vi "prepost.vi"(6 "What to call":enum16{"nothing", "pre-build", "post-build"}(ring), 7 "Post-build parameters":T1, 8 "error in (no error)":errorcluster, 11 "Build Parameters in":T2={"Build File"=path "", "File Format Version"=0, "Build Parameters v0.0"={"Project Root"=path "", "Build Root"=path "", "Source Root"=path "", "Namespace"="", "Overwrite Existing Files?"=FALSE, "Top Level VIs"=[], "Dynamic VIs"=[], "Exclude Lib Dirs from Build (None)"=[], "Destinations"=[]}, "Extra Parameters v1.0"={"Log File"=path "", "Include Hidden VIs"=FALSE, "Include Help Files"=FALSE, "Help File Dir"=path "", "Include Shared Libs"=TRUE, "Shared Lib Dir"=path "", "Include External Subrs"=TRUE, "External Subr Dir"=path "", "Support Files"=[], "EXE Icon File"=path "", "NewBuildRootDir"=FALSE, "UnsavedChangesMsgBox"=FALSE, "Ambiguous VIs Dest Dir"=path "", "Pre-build VI"=path "", "Post-build VI"=path "", "Revision File"=path "", "Version VI Name"="", "Version Ctrl Name"="", "Default Password"="", "RemovePolyVIsAndTDs"=FALSE, "Call-Back VIs"=[], "Allow CBVI & BH overlap"=FALSE, "Namespace convention"=enum."OpenG (suffix)", "Exe.AppFlags"=0, "Exe.LVRT Res Flags"=0}, "VI Property Specs"=[]} {"File Format Version" format="%.0x"; "Extra Parameters v1.0"."Exe.LVRT Res Flags" format="%.0x"; "Extra Parameters v1.0"."Exe.AppFlags" format="%.0x"}) -> (0 "error out":errorcluster, 1 "error type (fatal)":enum16{"fatal", "non-fatal", "warning"}(ring), 3 "Build Parameters in 2":T2={"Build File"=path "", "File Format Version"=0, "Build Parameters v0.0"={"Project Root"=path "", "Build Root"=path "", "Source Root"=path "", "Namespace"="", "Overwrite Existing Files?"=FALSE, "Top Level VIs"=[], "Dynamic VIs"=[], "Exclude Lib Dirs from Build (None)"=[], "Destinations"=[]}, "Extra Parameters v1.0"={"Log File"=path "", "Include Hidden VIs"=FALSE, "Include Help Files"=FALSE, "Help File Dir"=path "", "Include Shared Libs"=TRUE, "Shared Lib Dir"=path "", "Include External Subrs"=TRUE, "External Subr Dir"=path "", "Support Files"=[], "EXE Icon File"=path "", "NewBuildRootDir"=FALSE, "UnsavedChangesMsgBox"=FALSE, "Ambiguous VIs Dest Dir"=path "", "Pre-build VI"=path "", "Post-build VI"=path "", "Revision File"=path "", "Version VI Name"="", "Version Ctrl Name"="", "Default Password"="", "RemovePolyVIsAndTDs"=FALSE, "Call-Back VIs"=[], "Allow CBVI & BH overlap"=FALSE, "Namespace convention"=enum."OpenG (suffix)", "Exe.AppFlags"=0, "Exe.LVRT Res Flags"=0}, "VI Property Specs"=[]} {"File Format Version" format="%.0x"; "Extra Parameters v1.0"."Exe.LVRT Res Flags" format="%.0x"; "Extra Parameters v1.0"."Exe.AppFlags" format="%.0x"})   [LabVIEW 2009]
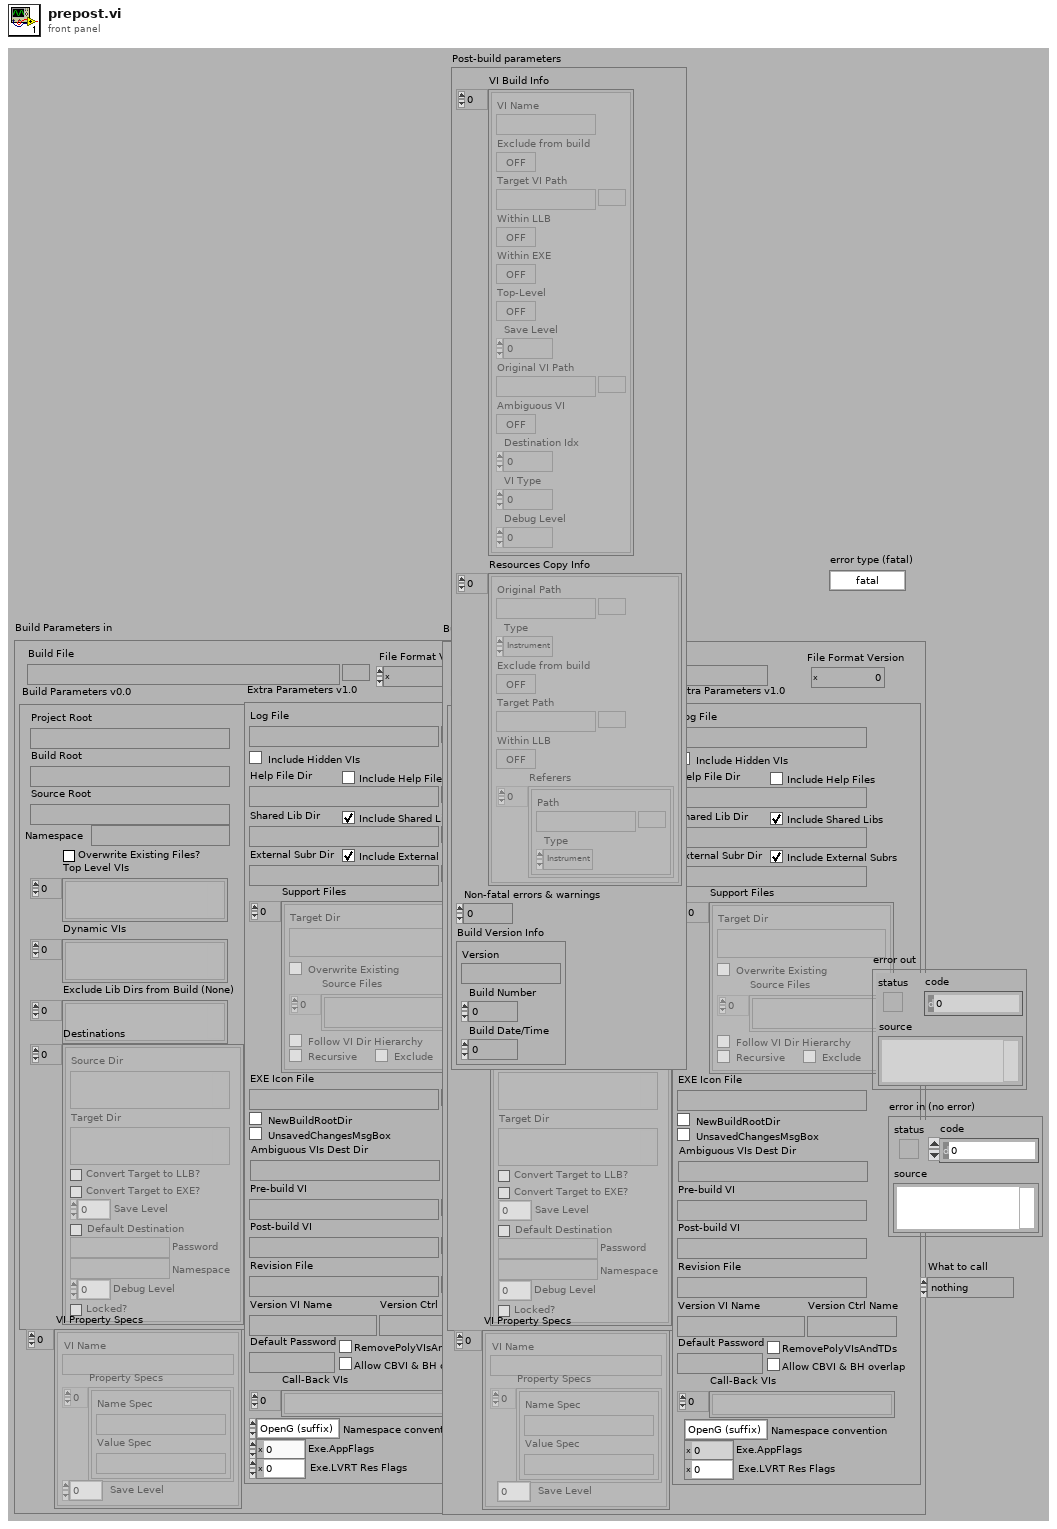
[diagram p1: front panel]
types:
  T1 = cluster{"VI Build Info":cluster{"VI Name":string, "Exclude from build":bool, "Target VI Path":path, "Within LLB":bool, "Within EXE":bool, "Top-Level":bool, "Save Level":i32, "Original VI Path":path, "Ambiguous VI":bool, "Destination Idx":i32, "VI Type":u32, "Debug Level":i32}[], "Resources Copy Info":cluster{"Original Path":path, "Type":enum32{"Instrument", "Control", "CIN", "External subroutine", "Shared library", "Run-time menu", "Help file", "Palette menu", "Polymorphic VI", "Library", "Library (10)"}, "Exclude from build":bool, "Target Path":path, "Within LLB":bool, "Referers":cluster{"Path":path, "Type":enum32{"Instrument", "Control", "CIN", "External subroutine", "Shared library", "Run-time menu", "Help file", "Palette menu", "Polymorphic VI", "Library", "Library (10)"}}[]}[], "Non-fatal errors & warnings":i32, "Build Version Info":cluster{"Version":string, "Build Number":u32, "Build Date/Time":dbl}}
  T2 = cluster{"Build File":path, "File Format Version":u32, "Build Parameters v0.0":cluster{"Project Root":path, "Build Root":path, "Source Root":path, "Namespace":string, "Overwrite Existing Files?":bool, "Top Level VIs":path[], "Dynamic VIs":path[], "Exclude Lib Dirs from Build (None)":path[], "Destinations":cluster{"Source Dir":path, "Target Dir":path, "Convert Target to LLB?":bool, "Convert Target to EXE?":bool, "Save Level":i32, "Default Destination":bool, "Password":string, "Namespace":string, "Debug Level":i32, "Locked?":bool}[]}, "Extra Parameters v1.0":cluster{"Log File":path, "Include Hidden VIs":bool, "Include Help Files":bool, "Help File Dir":path, "Include Shared Libs":bool, "Shared Lib Dir":path, "Include External Subrs":bool, "External Subr Dir":path, "Support Files":cluster{"Target Dir":path, "Overwrite Existing":bool, "Source Files":path[], "Follow VI Dir Hierarchy":bool, "Recursive":bool, "Exclude":bool}[], "EXE Icon File":path, "NewBuildRootDir":bool, "UnsavedChangesMsgBox":bool, "Ambiguous VIs Dest Dir":path, "Pre-build VI":path, "Post-build VI":path, "Revision File":path, "Version VI Name":string, "Version Ctrl Name":string, "Default Password":string, "RemovePolyVIsAndTDs":bool, "Call-Back VIs":path[], "Allow CBVI & BH overlap":bool, "Namespace convention":enum32{"OpenG (suffix)", "prefix", "prefix w space", "suffix"}, "Exe.AppFlags":u32, "Exe.LVRT Res Flags":i32}, "VI Property Specs":cluster{"VI Name":string, "Property Specs":cluster{"Name Spec":string, "Value Spec":string}[], "Save Level":i32}[]}
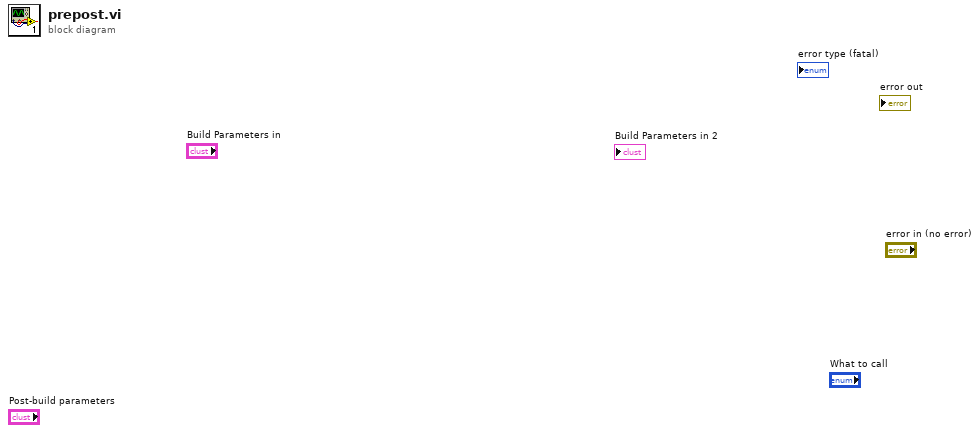
[diagram p0: block diagram]
diagram:
